vi "NI 5751 Multi Record Digital Trigger (Host).vi"() -> ()   [LabVIEW 2012] (continued)
2288.0, 5312.0, 7920.0, 9952.0, 11504.0, 12448.0, 12720.0, 12336.0, 11280.0, 9504.0, 7168.0, 4416.0, 1376.0, -1792.0, -4880.0, -7664.0, -9616.0, -10800.0, -11632.0, -12320.0, -12768.0, -12640.0, -11440.0, -9376.0, -6912.0, -4064.0, -1008.0, 2080.0, 5088.0, 7728.0, 9840.0, 11408.0, 12416.0, 12720.0, 12416.0, 11408.0, 9664.0, 7376.0, 4624.0, 1664.0, -1520.0, -4624.0, -7456.0, -9456.0, -10688.0, -11552.0, -12272.0, -12736.0, -12688.0, -11648.0, -9616.0, -7104.0, -4320.0, -1296.0, 1792.0, 4848.0, 7488.0, 9648.0, 11248.0, 12320.0, 12704.0, 12432.0, 11472.0, 9824.0, 7584.0, 4864.0, 1904.0, -1216.0, -4368.0, -7248.0, -9360.0, -10640.0, -11504.0, -12224.0, -12704.0, -12704.0, -11648.0, -9680.0, -7248.0, -4496.0, -1472.0, 1648.0, 4688.0, 7392.0, 9568.0, 11216.0, 12320.0, 12704.0, 12496.0, 11584.0, 9952.0, 7744.0, 5024.0, 2064.0, -1072.0, -4208.0, -7120.0, -9264.0]}, {"absoluteInitialX"=0.0, "xIncrement"=1.0, "wfm"=[-4672.0, -1712.0, 1376.0, 4464.0, 7184.0, 9392.0, 11088.0, 12240.0, 12720.0, 12528.0, 11696.0, 10128.0, 7984.0, 5360.0, 2400.0, -720.0, -3872.0, -6848.0, -9072.0, -10432.0, -11344.0, -12096.0, -12656.0, -12768.0, -11952.0, -10144.0, -7712.0, -4928.0, -1984.0, 1104.0, 4160.0, 6960.0, 9200.0, 10944.0, 12160.0, 12704.0, 12576.0, 11792.0, 10288.0, 8112.0, 5552.0, 2592.0, -528.0, -3664.0, -6672.0, -8976.0, -10384.0, -11312.0, -12048.0, -12624.0, -12768.0, -12032.0, -10224.0, -7792.0, -5072.0, -2128.0, 944.0, 4048.0, 6880.0, 9120.0, 10928.0, 12144.0, 12704.0, 12608.0, 11856.0, 10384.0, 8240.0, 5744.0, 2848.0, -288.0, -3472.0, -6512.0, -8832.0, -10304.0, -11248.0, -12000.0, -12576.0, -12752.0, -12096.0, -10336.0, -7968.0, -5248.0, -2352.0, 736.0, 3824.0, 6672.0, 9008.0, 10800.0, 12080.0, 12704.0, 12704.0, 12064.0, 10656.0, 8640.0, 6096.0, 3168.0, 112.0, -2992.0, -6032.0, -8528.0]}, {"absoluteInitialX"=0.0, "xIncrement"=1.0, "wfm"=[-2768.0, 272.0, 3392.0, 6288.0, 8672.0, 10576.0, 11920.0, 12688.0, 12720.0, 12128.0, 10848.0, 8896.0, 6416.0, 3584.0, 480.0, -2688.0, -5760.0, -8320.0, -9984.0, -11008.0, -11792.0, -12448.0, -12736.0, -12320.0, -10816.0, -8576.0, -5888.0, -2976.0, 32.0, 3088.0, 6048.0, 8512.0, 10448.0, 11872.0, 12624.0, 12736.0, 12176.0, 10944.0, 8960.0, 6544.0, 3712.0, 592.0, -2496.0, -5600.0, -8240.0, -9920.0, -10976.0, -11760.0, -12432.0, -12752.0, -12400.0, -10928.0, -8720.0, -6096.0, -3232.0, -224.0, 2928.0, 5904.0, 8400.0, 10320.0, 11760.0, 12576.0, 12768.0, 12256.0, 11056.0, 9136.0, 6704.0, 3920.0, 832.0, -2320.0, -5392.0, -8096.0, -9824.0, -10912.0, -11744.0, -12400.0, -12752.0, -12464.0, -11088.0, -8928.0, -6272.0, -3408.0, -416.0, 2720.0, 5728.0, 8208.0, 10224.0, 11680.0, 12576.0, 12768.0, 12336.0, 11216.0, 9376.0, 7008.0, 4240.0, 1216.0, -2016.0, -5072.0, -7824.0, -9664.0]}, {"absoluteInitialX"=0.0, "xIncrement"=1.0, "wfm"=[-3632.0, -624.0, 2480.0, 5488.0, 8080.0, 10128.0, 11616.0, 12560.0, 12800.0, 12368.0, 11280.0, 9504.0, 7120.0, 4416.0, 1376.0, -1776.0, -4864.0, -7712.0, -9584.0, -10752.0, -11584.0, -12272.0, -12688.0, -12560.0, -11360.0, -9296.0, -6736.0, -3888.0, -864.0, 2224.0, 5280.0, 7888.0, 9968.0, 11504.0, 12496.0, 12768.0, 12416.0, 11376.0, 9664.0, 7280.0, 4592.0, 1536.0, -1600.0, -4704.0, -7536.0, -9504.0, -10704.0, -11520.0, -12240.0, -12688.0, -12608.0, -11456.0, -9456.0, -6896.0, -4064.0, -1056.0, 2064.0, 5088.0, 7664.0, 9776.0, 11408.0, 12432.0, 12768.0, 12448.0, 11424.0, 9744.0, 7456.0, 4768.0, 1776.0, -1344.0, -4512.0, -7360.0, -9392.0, -10656.0, -11504.0, -12224.0, -12672.0, -12656.0, -11600.0, -9600.0, -7056.0, -4272.0, -1264.0, 1808.0, 4848.0, 7552.0, 9680.0, 11312.0, 12400.0, 12752.0, 12480.0, 11520.0, 9824.0, 7520.0, 4848.0, 1904.0, -1280.0, -4416.0, -7280.0, -9328.0]}, {"absoluteInitialX"=0.0, "xIncrement"=1.0, "wfm"=[-4400.0, -1424.0, 1712.0, 4720.0, 7408.0, 9600.0, 11248.0, 12320.0, 12736.0, 12528.0, 11568.0, 9968.0, 7760.0, 5056.0, 2096.0, -1040.0, -4192.0, -7120.0, -9264.0, -10544.0, -11424.0, -12176.0, -12672.0, -12704.0, -11792.0, -9920.0, -7440.0, -4672.0, -1696.0, 1392.0, 4416.0, 7184.0, 9440.0, 11136.0, 12240.0, 12704.0, 12528.0, 11648.0, 10064.0, 7904.0, 5248.0, 2256.0, -832.0, -4000.0, -6928.0, -9152.0, -10512.0, -11392.0, -12128.0, -12656.0, -12752.0, -11872.0, -10000.0, -7552.0, -4800.0, -1808.0, 1280.0, 4288.0, 7088.0, 9312.0, 11040.0, 12224.0, 12704.0, 12544.0, 11712.0, 10176.0, 8032.0, 5360.0, 2448.0, -656.0, -3792.0, -6768.0, -9040.0, -10432.0, -11344.0, -12112.0, -12656.0, -12768.0, -12016.0, -10192.0, -7792.0, -5040.0, -2096.0, 976.0, 4048.0, 6912.0, 9152.0, 10896.0, 12144.0, 12720.0, 12608.0, 11856.0, 10384.0, 8208.0, 5648.0, 2752.0, -320.0, -3520.0, -6544.0, -8880.0]}, {"absoluteInitialX"=0.0, "xIncrement"=1.0, "wfm"=[-2336.0, 720.0, 3824.0, 6672.0, 8976.0, 10784.0, 12064.0, 12672.0, 12624.0, 11952.0, 10480.0, 8432.0, 5840.0, 2944.0, -112.0, -3296.0, -6304.0, -8720.0, -10256.0, -11216.0, -11984.0, -12560.0, -12800.0, -12224.0, -10528.0, -8192.0, -5504.0, -2576.0, 448.0, 3520.0, 6448.0, 8800.0, 10640.0, 11968.0, 12656.0, 12624.0, 11984.0, 10624.0, 8608.0, 6064.0, 3216.0, 128.0, -3088.0, -6064.0, -8544.0, -10144.0, -11152.0, -11936.0, -12544.0, -12816.0, -12304.0, -10720.0, -8400.0, -5744.0, -2816.0, 192.0, 3296.0, 6192.0, 8624.0, 10512.0, 11888.0, 12608.0, 12688.0, 12096.0, 10800.0, 8832.0, 6400.0, 3568.0, 480.0, -2672.0, -5824.0, -8368.0, -10016.0, -11040.0, -11856.0, -12480.0, -12800.0, -12400.0, -10880.0, -8688.0, -6016.0, -3104.0, -96.0, 3024.0, 5984.0, 8432.0, 10368.0, 11808.0, 12592.0, 12704.0, 12192.0, 10944.0, 9040.0, 6592.0, 3840.0, 768.0, -2416.0, -5504.0, -8160.0, -9904.0]}, {"absoluteInitialX"=0.0, "xIncrement"=1.0, "wfm"=[-3296.0, -288.0, 2784.0, 5728.0, 8224.0, 10224.0, 11696.0, 12576.0, 12720.0, 12224.0, 11040.0, 9200.0, 6800.0, 3968.0, 912.0, -2224.0, -5264.0, -8000.0, -9808.0, -10896.0, -11712.0, -12384.0, -12784.0, -12528.0, -11200.0, -9024.0, -6416.0, -3552.0, -544.0, 2592.0, 5616.0, 8144.0, 10112.0, 11600.0, 12512.0, 12736.0, 12288.0, 11168.0, 9376.0, 6976.0, 4240.0, 1216.0, -1968.0, -5072.0, -7840.0, -9696.0, -10832.0, -11664.0, -12336.0, -12768.0, -12576.0, -11264.0, -9184.0, -6688.0, -3824.0, -800.0, 2352.0, 5408.0, 7936.0, 9968.0, 11520.0, 12448.0, 12704.0, 12352.0, 11248.0, 9488.0, 7216.0, 4464.0, 1440.0, -1680.0, -4816.0, -7632.0, -9568.0, -10752.0, -11600.0, -12288.0, -12736.0, -12640.0, -11456.0, -9392.0, -6864.0, -4048.0, -1008.0, 2048.0, 5056.0, 7712.0, 9840.0, 11408.0, 12448.0, 12720.0, 12384.0, 11408.0, 9712.0, 7392.0, 4672.0, 1680.0, -1456.0, -4592.0, -7424.0, -9440.0]}, {"absoluteInitialX"=0.0, "xIncrement"=1.0, "wfm"=[-4272.0, -1264.0, 1808.0, 4816.0, 7520.0, 9680.0, 11280.0, 12352.0, 12704.0, 12464.0, 11520.0, 9840.0, 7600.0, 4944.0, 1920.0, -1184.0, -4352.0, -7232.0, -9296.0, -10608.0, -11472.0, -12192.0, -12704.0, -12720.0, -11744.0, -9808.0, -7344.0, -4528.0, -1568.0, 1520.0, 4592.0, 7344.0, 9520.0, 11168.0, 12288.0, 12720.0, 12496.0, 11600.0, 9984.0, 7744.0, 5088.0, 2128.0, -976.0, -4112.0, -7040.0, -9216.0, -10544.0, -11440.0, -12176.0, -12688.0, -12768.0, -11904.0, -9952.0, -7552.0, -4768.0, -1808.0, 1328.0, 4384.0, 7104.0, 9328.0, 11024.0, 12208.0, 12688.0, 12512.0, 11680.0, 10128.0, 7968.0, 5296.0, 2384.0, -752.0, -3872.0, -6832.0, -9072.0, -10464.0, -11392.0, -12128.0, -12640.0, -12800.0, -11984.0, -10128.0, -7728.0, -5008.0, -2048.0, 1040.0, 4128.0, 6928.0, 9200.0, 10944.0, 12144.0, 12704.0, 12592.0, 11808.0, 10304.0, 8176.0, 5616.0, 2704.0, -400.0, -3552.0, -6592.0, -8912.0]}, {"absoluteInitialX"=0.0, "xIncrement"=1.0, "wfm"=[-2336.0, 656.0, 3776.0, 6640.0, 8976.0, 10784.0, 12032.0, 12656.0, 12608.0, 11888.0, 10512.0, 8448.0, 5856.0, 2992.0, -96.0, -3248.0, -6256.0, -8704.0, -10240.0, -11216.0, -11984.0, -12576.0, -12784.0, -12208.0, -10560.0, -8240.0, -5552.0, -2624.0, 448.0, 3552.0, 6496.0, 8832.0, 10672.0, 11968.0, 12640.0, 12656.0, 11984.0, 10592.0, 8544.0, 6064.0, 3184.0, 80.0, -3024.0, -6064.0, -8608.0, -10160.0, -11152.0, -11904.0, -12528.0, -12800.0, -12320.0, -10704.0, -8432.0, -5744.0, -2800.0, 272.0, 3392.0, 6288.0, 8640.0, 10528.0, 11904.0, 12624.0, 12672.0, 12112.0, 10832.0, 8832.0, 6352.0, 3488.0, 400.0, -2752.0, -5776.0, -8368.0, -10032.0, -11072.0, -11856.0, -12464.0, -12800.0, -12400.0, -10928.0, -8688.0, -6032.0, -3136.0, -96.0, 3008.0, 5984.0, 8416.0, 10368.0, 11792.0, 12560.0, 12672.0, 12160.0, 10944.0, 9024.0, 6576.0, 3760.0, 704.0, -2496.0, -5568.0, -8224.0, -9952.0]}, {"absoluteInitialX"=0.0, "xIncrement"=1.0, "wfm"=[-3376.0, -336.0, 2816.0, 5744.0, 8272.0, 10256.0, 11696.0, 12560.0, 12704.0, 12240.0, 11056.0, 9200.0, 6736.0, 4000.0, 944.0, -2208.0, -5328.0, -8048.0, -9840.0, -10912.0, -11728.0, -12400.0, -12800.0, -12544.0, -11200.0, -9056.0, -6464.0, -3600.0, -544.0, 2528.0, 5536.0, 8064.0, 10112.0, 11600.0, 12496.0, 12704.0, 12288.0, 11200.0, 9392.0, 7040.0, 4256.0, 1280.0, -1920.0, -5024.0, -7792.0, -9664.0, -10800.0, -11664.0, -12352.0, -12768.0, -12608.0, -11328.0, -9200.0, -6624.0, -3808.0, -768.0, 2288.0, 5296.0, 7872.0, 9952.0, 11536.0, 12480.0, 12752.0, 12384.0, 11312.0, 9552.0, 7200.0, 4480.0, 1472.0, -1632.0, -4832.0, -7648.0, -9584.0, -10752.0, -11600.0, -12288.0, -12736.0, -12624.0, -11472.0, -9424.0, -6848.0, -4016.0, -1008.0, 2112.0, 5120.0, 7760.0, 9872.0, 11424.0, 12432.0, 12752.0, 12384.0, 11344.0, 9632.0, 7280.0, 4560.0, 1584.0, -1568.0, -4704.0, -7552.0, -9504.0]}, {"absoluteInitialX"=0.0, "xIncrement"=1.0, "wfm"=[-4032.0, -1104.0, 1968.0, 4976.0, 7632.0, 9776.0, 11360.0, 12400.0, 12720.0, 12384.0, 11376.0, 9680.0, 7392.0, 4672.0, 1712.0, -1456.0, -4560.0, -7440.0, -9472.0, -10688.0, -11552.0, -12256.0, -12720.0, -12704.0, -11632.0, -9632.0, -7120.0, -4288.0, -1280.0, 1776.0, 4816.0, 7536.0, 9648.0, 11264.0, 12352.0, 12704.0, 12448.0, 11504.0, 9888.0, 7664.0, 4992.0, 1984.0, -1152.0, -4240.0, -7168.0, -9296.0, -10592.0, -11472.0, -12192.0, -12688.0, -12736.0, -11760.0, -9776.0, -7360.0, -4544.0, -1616.0, 1504.0, 4560.0, 7248.0, 9472.0, 11120.0, 12288.0, 12688.0, 12496.0, 11616.0, 10000.0, 7792.0, 5136.0, 2176.0, -1008.0, -4128.0, -7056.0, -9216.0, -10560.0, -11440.0, -12160.0, -12688.0, -12736.0, -11840.0, -9984.0, -7520.0, -4736.0, -1808.0, 1280.0, 4368.0, 7136.0, 9360.0, 11088.0, 12224.0, 12688.0, 12528.0, 11712.0, 10144.0, 8032.0, 5392.0, 2368.0, -768.0, -3904.0, -6832.0, -9072.0]}, {"absoluteInitialX"=0.0, "xIncrement"=1.0, "wfm"=[-2000.0, 1120.0, 4176.0, 6960.0, 9216.0, 10960.0, 12176.0, 12720.0, 12576.0, 11808.0, 10336.0, 8240.0, 5568.0, 2656.0, -464.0, -3600.0, -6608.0, -8912.0, -10336.0, -11280.0, -12048.0, -12608.0, -12768.0, -12048.0, -10272.0, -7888.0, -5184.0, -2208.0, 864.0, 3952.0, 6784.0, 9088.0, 10832.0, 12096.0, 12640.0, 12592.0, 11856.0, 10384.0, 8288.0, 5744.0, 2848.0, -272.0, -3424.0, -6448.0, -8816.0, -10304.0, -11248.0, -12000.0, -12608.0, -12800.0, -12160.0, -10448.0, -8112.0, -5408.0, -2448.0, 608.0, 3712.0, 6560.0, 8880.0, 10736.0, 12016.0, 12672.0, 12640.0, 11984.0, 10608.0, 8528.0, 6000.0, 3184.0, 112.0, -3088.0, -6144.0, -8592.0, -10160.0, -11152.0, -11920.0, -12528.0, -12816.0, -12288.0, -10688.0, -8416.0, -5696.0, -2784.0, 272.0, 3360.0, 6304.0, 8688.0, 10544.0, 11920.0, 12624.0, 12672.0, 12096.0, 10800.0, 8848.0, 6384.0, 3536.0, 480.0, -2704.0, -5760.0, -8336.0, -10016.0]}, {"absoluteInitialX"=0.0, "xIncrement"=1.0, "wfm"=[-3152.0, -112.0, 3056.0, 5968.0, 8400.0, 10384.0, 11776.0, 12576.0, 12688.0, 12160.0, 10928.0, 9056.0, 6576.0, 3744.0, 640.0, -2480.0, -5584.0, -8224.0, -9920.0, -10976.0, -11776.0, -12432.0, -12800.0, -12496.0, -11072.0, -8864.0, -6256.0, -3392.0, -368.0, 2768.0, 5744.0, 8288.0, 10240.0, 11664.0, 12544.0, 12688.0, 12208.0, 11024.0, 9104.0, 6688.0, 3936.0, 880.0, -2304.0, -5376.0, -8048.0, -9856.0, -10928.0, -11744.0, -12432.0, -12816.0, -12544.0, -11232.0, -9104.0, -6464.0, -3584.0, -576.0, 2528.0, 5520.0, 8048.0, 10080.0, 11584.0, 12496.0, 12704.0, 12288.0, 11152.0, 9328.0, 6976.0, 4144.0, 1120.0, -1984.0, -5104.0, -7872.0, -9728.0, -10864.0, -11696.0, -12368.0, -12800.0, -12608.0, -11376.0, -9232.0, -6672.0, -3856.0, -848.0, 2240.0, 5264.0, 7856.0, 9920.0, 11456.0, 12416.0, 12688.0, 12320.0, 11232.0, 9520.0, 7168.0, 4400.0, 1408.0, -1696.0, -4800.0, -7632.0, -9600.0]}, {"absoluteInitialX"=0.0, "xIncrement"=1.0, "wfm"=[-4080.0, -1056.0, 2048.0, 5056.0, 7696.0, 9840.0, 11392.0, 12400.0, 12704.0, 12368.0, 11360.0, 9648.0, 7344.0, 4624.0, 1616.0, -1504.0, -4672.0, -7504.0, -9504.0, -10704.0, -11584.0, -12288.0, -12752.0, -12704.0, -11616.0, -9632.0, -7120.0, -4240.0, -1248.0, 1840.0, 4848.0, 7520.0, 9664.0, 11264.0, 12336.0, 12720.0, 12432.0, 11440.0, 9760.0, 7504.0, 4800.0, 1808.0, -1280.0, -4416.0, -7360.0, -9376.0, -10640.0, -11536.0, -12256.0, -12752.0, -12736.0, -11712.0, -9760.0, -7280.0, -4480.0, -1488.0, 1584.0, 4608.0, 7328.0, 9504.0, 11152.0, 12288.0, 12736.0, 12496.0, 11584.0, 10016.0, 7840.0, 5168.0, 2224.0, -960.0, -4128.0, -7040.0, -9184.0, -10528.0, -11408.0, -12160.0, -12688.0, -12768.0, -11856.0, -9968.0, -7504.0, -4688.0, -1728.0, 1344.0, 4400.0, 7200.0, 9376.0, 11056.0, 12240.0, 12720.0, 12528.0, 11728.0, 10176.0, 7984.0, 5344.0, 2432.0, -624.0, -3808.0, -6784.0, -9024.0]}, {"absoluteInitialX"=0.0, "xIncrement"=1.0, "wfm"=[-2016.0, 1008.0, 4096.0, 6880.0, 9168.0, 10928.0, 12160.0, 12736.0, 12640.0, 11904.0, 10496.0, 8416.0, 5808.0, 2896.0, -208.0, -3344.0, -6352.0, -8768.0, -10256.0, -11184.0, -11952.0, -12544.0, -12752.0, -12128.0, -10464.0, -8128.0, -5424.0, -2528.0, 608.0, 3680.0, 6544.0, 8880.0, 10736.0, 12016.0, 12704.0, 12672.0, 12016.0, 10656.0, 8592.0, 6080.0, 3216.0, 128.0, -3024.0, -6032.0, -8544.0, -10128.0, -11104.0, -11904.0, -12512.0, -12752.0, -12208.0, -10624.0, -8320.0, -5632.0, -2704.0, 320.0, 3424.0, 6336.0, 8752.0, 10608.0, 11936.0, 12688.0, 12704.0, 12096.0, 10752.0, 8784.0, 6352.0, 3456.0, 336.0, -2816.0, -5824.0, -8368.0, -10032.0, -11056.0, -11824.0, -12464.0, -12784.0, -12336.0, -10832.0, -8528.0, -5904.0, -3008.0, 16.0, 3168.0, 6080.0, 8544.0, 10448.0, 11856.0, 12624.0, 12720.0, 12176.0, 10880.0, 8960.0, 6512.0, 3648.0, 544.0, -2592.0, -5664.0, -8288.0, -9968.0]}, {"absoluteInitialX"=0.0, "xIncrement"=1.0, "wfm"=[-3136.0, -160.0, 2944.0, 5936.0, 8416.0, 10352.0, 11776.0, 12608.0, 12720.0, 12208.0, 10960.0, 9056.0, 6608.0, 3808.0, 752.0, -2416.0, -5504.0, -8144.0, -9904.0, -10976.0, -11776.0, -12400.0, -12784.0, -12432.0, -11008.0, -8848.0, -6192.0, -3296.0, -272.0, 2848.0, 5792.0, 8256.0, 10272.0, 11712.0, 12560.0, 12736.0, 12272.0, 11072.0, 9232.0, 6832.0, 4016.0, 992.0, -2176.0, -5264.0, -7968.0, -9776.0, -10880.0, -11680.0, -12368.0, -12768.0, -12544.0, -11216.0, -9088.0, -6496.0, -3632.0, -608.0, 2512.0, 5488.0, 8064.0, 10096.0, 11616.0, 12528.0, 12704.0, 12272.0, 11216.0, 9424.0, 7056.0, 4272.0, 1248.0, -1936.0, -5008.0, -7792.0, -9648.0, -10816.0, -11632.0, -12336.0, -12752.0, -12576.0, -11328.0, -9280.0, -6688.0, -3808.0, -800.0, 2304.0, 5280.0, 7872.0, 9984.0, 11504.0, 12480.0, 12704.0, 12336.0, 11264.0, 9488.0, 7104.0, 4368.0, 1360.0, -1840.0, -4960.0, -7712.0, -9648.0]}, {"absoluteInitialX"=0.0, "xIncrement"=1.0, "wfm"=[-3968.0, -944.0, 2144.0, 5152.0, 7776.0, 9856.0, 11424.0, 12432.0, 12720.0, 12368.0, 11328.0, 9568.0, 7280.0, 4576.0, 1568.0, -1568.0, -4704.0, -7520.0, -9520.0, -10752.0, -11584.0, -12288.0, -12752.0, -12688.0, -11552.0, -9504.0, -7024.0, -4240.0, -1216.0, 1920.0, 4944.0, 7600.0, 9728.0, 11344.0, 12368.0, 12720.0, 12432.0, 11424.0, 9744.0, 7488.0, 4800.0, 1824.0, -1360.0, -4480.0, -7344.0, -9408.0, -10656.0, -11520.0, -12224.0, -12720.0, -12704.0, -11664.0, -9696.0, -7232.0, -4416.0, -1392.0, 1680.0, 4704.0, 7376.0, 9552.0, 11248.0, 12336.0, 12736.0, 12464.0, 11552.0, 9904.0, 7712.0, 5056.0, 2080.0, -1088.0, -4208.0, -7120.0, -9280.0, -10576.0, -11456.0, -12160.0, -12688.0, -12752.0, -11824.0, -9920.0, -7440.0, -4704.0, -1728.0, 1376.0, 4448.0, 7152.0, 9376.0, 11104.0, 12240.0, 12704.0, 12544.0, 11632.0, 10048.0, 7872.0, 5168.0, 2240.0, -848.0, -4016.0, -6992.0, -9184.0]}, {"absoluteInitialX"=0.0, "xIncrement"=1.0, "wfm"=[-4912.0, -1920.0, 1168.0, 4224.0, 7040.0, 9280.0, 10992.0, 12192.0, 12656.0, 12528.0, 11728.0, 10208.0, 8064.0, 5408.0, 2480.0, -640.0, -3776.0, -6720.0, -9024.0, -10448.0, -11328.0, -12112.0, -12656.0, -12800.0, -12016.0, -10176.0, -7824.0, -5040.0, -2064.0, 976.0, 4032.0, 6896.0, 9184.0, 10928.0, 12128.0, 12656.0, 12544.0, 11744.0, 10304.0, 8112.0, 5504.0, 2560.0, -528.0, -3664.0, -6656.0, -8992.0, -10400.0, -11312.0, -12080.0, -12640.0, -12784.0, -12064.0, -10272.0, -7888.0, -5168.0, -2208.0, 864.0, 3936.0, 6752.0, 9088.0, 10832.0, 12080.0, 12656.0, 12560.0, 11824.0, 10352.0, 8256.0, 5664.0, 2768.0, -416.0, -3536.0, -6528.0, -8864.0, -10352.0, -11296.0, -12048.0, -12608.0, -12800.0, -12144.0, -10384.0, -8032.0, -5280.0, -2336.0, 736.0, 3824.0, 6640.0, 8944.0, 10768.0, 12048.0, 12672.0, 12640.0, 11968.0, 10608.0, 8544.0, 5952.0, 3120.0, 32.0, -3120.0, -6192.0, -8656.0]}, {"absoluteInitialX"=0.0, "xIncrement"=1.0, "wfm"=[-2672.0, 368.0, 3472.0, 6352.0, 8736.0, 10656.0, 11968.0, 12672.0, 12672.0, 12112.0, 10816.0, 8720.0, 6240.0, 3440.0, 352.0, -2752.0, -5840.0, -8400.0, -10032.0, -11040.0, -11840.0, -12448.0, -12768.0, -12320.0, -10784.0, -8592.0, -5904.0, -2992.0, 48.0, 3120.0, 6064.0, 8512.0, 10448.0, 11824.0, 12608.0, 12672.0, 12144.0, 10880.0, 8960.0, 6512.0, 3632.0, 544.0, -2688.0, -5728.0, -8304.0, -9984.0, -11024.0, -11808.0, -12448.0, -12784.0, -12400.0, -10912.0, -8704.0, -6032.0, -3168.0, -144.0, 2928.0, 5888.0, 8368.0, 10320.0, 11744.0, 12576.0, 12752.0, 12272.0, 11040.0, 9168.0, 6784.0, 3968.0, 896.0, -2240.0, -5344.0, -8064.0, -9824.0, -10912.0, -11728.0, -12384.0, -12768.0, -12480.0, -11152.0, -8992.0, -6352.0, -3472.0, -464.0, 2672.0, 5600.0, 8160.0, 10160.0, 11664.0, 12544.0, 12752.0, 12288.0, 11120.0, 9328.0, 6912.0, 4112.0, 1088.0, -1984.0, -5136.0, -7872.0, -9712.0]}, {"absoluteInitialX"=0.0, "xIncrement"=1.0, "wfm"=[-3680.0, -656.0, 2464.0, 5408.0, 7984.0, 10064.0, 11568.0, 12544.0, 12752.0, 12384.0, 11248.0, 9456.0, 7120.0, 4320.0, 1312.0, -1824.0, -4976.0, -7760.0, -9648.0, -10784.0, -11616.0, -12320.0, -12752.0, -12624.0, -11408.0, -9296.0, -6784.0, -3984.0, -960.0, 2176.0, 5168.0, 7824.0, 9920.0, 11440.0, 12432.0, 12720.0, 12352.0, 11328.0, 9552.0, 7216.0, 4512.0, 1472.0, -1616.0, -4752.0, -7632.0, -9536.0, -10736.0, -11584.0, -12288.0, -12736.0, -12672.0, -11520.0, -9456.0, -6928.0, -4144.0, -1152.0, 1968.0, 5024.0, 7632.0, 9776.0, 11344.0, 12384.0, 12736.0, 12416.0, 11408.0, 9744.0, 7440.0, 4688.0, 1680.0, -1440.0, -4592.0, -7440.0, -9440.0, -10688.0, -11536.0, -12240.0, -12720.0, -12688.0, -11632.0, -9632.0, -7136.0, -4336.0, -1360.0, 1760.0, 4784.0, 7488.0, 9648.0, 11232.0, 12352.0, 12704.0, 12416.0, 11456.0, 9792.0, 7520.0, 4816.0, 1856.0, -1280.0, -4416.0, -7296.0, -9376.0]}, {"absoluteInitialX"=0.0, "xIncrement"=1.0, "wfm"=[-4464.0, -1504.0, 1616.0, 4656.0, 7344.0, 9552.0, 11184.0, 12304.0, 12704.0, 12464.0, 11504.0, 9840.0, 7616.0, 5024.0, 2000.0, -1152.0, -4288.0, -7184.0, -9312.0, -10576.0, -11472.0, -12192.0, -12704.0, -12736.0, -11792.0, -9840.0, -7392.0, -4592.0, -1616.0, 1488.0, 4528.0, 7232.0, 9424.0, 11136.0, 12256.0, 12704.0, 12512.0, 11648.0, 10048.0, 7888.0, 5168.0, 2176.0, -944.0, -4048.0, -6976.0, -9184.0, -10512.0, -11392.0, -12144.0, -12672.0, -12768.0, -11888.0, -10032.0, -7648.0, -4880.0, -1840.0, 1248.0, 4288.0, 7088.0, 9312.0, 11024.0, 12208.0, 12688.0, 12544.0, 11712.0, 10192.0, 8016.0, 5456.0, 2512.0, -656.0, -3792.0, -6736.0, -9008.0, -10400.0, -11344.0, -12112.0, -12624.0, -12752.0, -12000.0, -10160.0, -7744.0, -5008.0, -2080.0, 960.0, 4064.0, 6880.0, 9184.0, 10944.0, 12144.0, 12704.0, 12624.0, 11888.0, 10448.0, 8336.0, 5760.0, 2816.0, -288.0, -3424.0, -6416.0, -8784.0]}, {"absoluteInitialX"=0.0, "xIncrement"=1.0, "wfm"=[-2384.0, 656.0, 3728.0, 6624.0, 8928.0, 10736.0, 12048.0, 12720.0, 12688.0, 12032.0, 10640.0, 8608.0, 6080.0, 3248.0, 176.0, -3024.0, -6032.0, -8528.0, -10112.0, -11104.0, -11856.0, -12496.0, -12736.0, -12240.0, -10640.0, -8320.0, -5648.0, -2784.0, 272.0, 3376.0, 6288.0, 8704.0, 10576.0, 11936.0, 12688.0, 12736.0, 12096.0, 10832.0, 8816.0, 6352.0, 3504.0, 416.0, -2736.0, -5840.0, -8368.0, -10000.0, -11008.0, -11808.0, -12448.0, -12752.0, -12304.0, -10800.0, -8560.0, -5856.0, -2976.0, 96.0, 3200.0, 6112.0, 8544.0, 10512.0, 11888.0, 12656.0, 12736.0, 12208.0, 10928.0, 9040.0, 6560.0, 3728.0, 672.0, -2512.0, -5584.0, -8192.0, -9888.0, -10944.0, -11760.0, -12400.0, -12736.0, -12400.0, -10960.0, -8736.0, -6128.0, -3232.0, -224.0, 2896.0, 5856.0, 8352.0, 10336.0, 11744.0, 12592.0, 12768.0, 12320.0, 11088.0, 9216.0, 6832.0, 4032.0, 944.0, -2192.0, -5328.0, -8016.0, -9792.0]}, {"absoluteInitialX"=0.0, "xIncrement"=1.0, "wfm"=[-3472.0, -464.0, 2688.0, 5664.0, 8160.0, 10192.0, 11664.0, 12576.0, 12752.0, 12272.0, 11104.0, 9280.0, 6864.0, 4096.0, 1024.0, -2144.0, -5216.0, -7920.0, -9744.0, -10848.0, -11648.0, -12352.0, -12736.0, -12512.0, -11184.0, -9040.0, -6464.0, -3648.0, -640.0, 2544.0, 5552.0, 8128.0, 10112.0, 11616.0, 12528.0, 12720.0, 12256.0, 11120.0, 9296.0, 6912.0, 4112.0, 1104.0, -2080.0, -5168.0, -7904.0, -9744.0, -10864.0, -11664.0, -12352.0, -12752.0, -12512.0, -11248.0, -9072.0, -6512.0, -3664.0, -592.0, 2512.0, 5472.0, 8016.0, 10080.0, 11584.0, 12528.0, 12736.0, 12336.0, 11200.0, 9392.0, 7024.0, 4176.0, 1184.0, -1952.0, -5056.0, -7776.0, -9664.0, -10800.0, -11664.0, -12336.0, -12752.0, -12560.0, -11296.0, -9216.0, -6640.0, -3776.0, -752.0, 2352.0, 5408.0, 7952.0, 10032.0, 11520.0, 12496.0, 12736.0, 12352.0, 11232.0, 9488.0, 7104.0, 4320.0, 1312.0, -1808.0, -4976.0, -7760.0, -9648.0]}, {"absoluteInitialX"=0.0, "xIncrement"=1.0, "wfm"=[-3888.0, -896.0, 2240.0, 5232.0, 7824.0, 9904.0, 11456.0, 12464.0, 12752.0, 12400.0, 11360.0, 9616.0, 7280.0, 4544.0, 1504.0, -1600.0, -4704.0, -7520.0, -9504.0, -10704.0, -11552.0, -12240.0, -12720.0, -12656.0, -11504.0, -9504.0, -6928.0, -4064.0, -1056.0, 2016.0, 5008.0, 7680.0, 9808.0, 11392.0, 12432.0, 12736.0, 12448.0, 11472.0, 9776.0, 7472.0, 4752.0, 1760.0, -1392.0, -4480.0, -7376.0, -9392.0, -10624.0, -11472.0, -12208.0, -12688.0, -12656.0, -11584.0, -9584.0, -7072.0, -4240.0, -1248.0, 1888.0, 4880.0, 7536.0, 9696.0, 11312.0, 12400.0, 12768.0, 12512.0, 11568.0, 9920.0, 7680.0, 4992.0, 2016.0, -1120.0, -4272.0, -7152.0, -9264.0, -10560.0, -11408.0, -12144.0, -12640.0, -12656.0, -11680.0, -9728.0, -7296.0, -4544.0, -1552.0, 1600.0, 4624.0, 7392.0, 9552.0, 11216.0, 12352.0, 12768.0, 12576.0, 11648.0, 10048.0, 7904.0, 5264.0, 2288.0, -864.0, -3952.0, -6896.0, -9104.0]}, {"absoluteInitialX"=0.0, "xIncrement"=1.0, "wfm"=[-4784.0, -1808.0, 1312.0, 4384.0, 7136.0, 9344.0, 11088.0, 12288.0, 12784.0, 12656.0, 11840.0, 10320.0, 8160.0, 5632.0, 2688.0, -448.0, -3568.0, -6592.0, -8864.0, -10304.0, -11232.0, -11952.0, -12560.0, -12704.0, -11984.0, -10208.0, -7808.0, -5056.0, -2144.0, 912.0, 4000.0, 6848.0, 9152.0, 10928.0, 12192.0, 12752.0, 12656.0, 11920.0, 10480.0, 8368.0, 5840.0, 2960.0, -144.0, -3280.0, -6336.0, -8736.0, -10208.0, -11184.0, -11952.0, -12512.0, -12736.0, -12080.0, -10416.0, -8016.0, -5280.0, -2368.0, 688.0, 3792.0, 6656.0, 8976.0, 10848.0, 12112.0, 12736.0, 12704.0, 12016.0, 10592.0, 8544.0, 5984.0, 3120.0, -32.0, -3152.0, -6160.0, -8608.0, -10160.0, -11104.0, -11904.0, -12496.0, -12720.0, -12160.0, -10496.0, -8160.0, -5488.0, -2592.0, 496.0, 3632.0, 6528.0, 8928.0, 10736.0, 12032.0, 12736.0, 12752.0, 12112.0, 10704.0, 8736.0, 6224.0, 3344.0, 272.0, -2912.0, -5920.0, -8448.0]}, {"absoluteInitialX"=0.0, "xIncrement"=1.0, "wfm"=[-2768.0, 288.0, 3392.0, 6336.0, 8736.0, 10592.0, 11952.0, 12688.0, 12752.0, 12144.0, 10816.0, 8848.0, 6352.0, 3456.0, 400.0, -2688.0, -5792.0, -8352.0, -9984.0, -10992.0, -11792.0, -12416.0, -12736.0, -12304.0, -10752.0, -8528.0, -5856.0, -2976.0, 48.0, 3168.0, 6112.0, 8560.0, 10496.0, 11888.0, 12656.0, 12736.0, 12192.0, 10928.0, 8992.0, 6544.0, 3712.0, 656.0, -2512.0, -5600.0, -8192.0, -9904.0, -10960.0, -11744.0, -12400.0, -12736.0, -12352.0, -10880.0, -8704.0, -6016.0, -3120.0, -96.0, 2992.0, 5968.0, 8448.0, 10400.0, 11824.0, 12640.0, 12784.0, 12304.0, 11104.0, 9184.0, 6736.0, 3952.0, 928.0, -2192.0, -5312.0, -8000.0, -9792.0, -10864.0, -11680.0, -12320.0, -12720.0, -12448.0, -11072.0, -8912.0, -6304.0, -3440.0, -416.0, 2720.0, 5728.0, 8208.0, 10240.0, 11712.0, 12608.0, 12784.0, 12352.0, 11232.0, 9408.0, 7008.0, 4256.0, 1216.0, -1968.0, -5072.0, -7808.0, -9632.0]}, {"absoluteInitialX"=0.0, "xIncrement"=1.0, "wfm"=[-3744.0, -752.0, 2368.0, 5392.0, 7968.0, 10016.0, 11568.0, 12528.0, 12768.0, 12384.0, 11328.0, 9568.0, 7232.0, 4464.0, 1472.0, -1712.0, -4800.0, -7648.0, -9520.0, -10720.0, -11568.0, -12256.0, -12704.0, -12592.0, -11408.0, -9312.0, -6832.0, -3984.0, -992.0, 2144.0, 5184.0, 7760.0, 9856.0, 11440.0, 12432.0, 12768.0, 12432.0, 11392.0, 9632.0, 7360.0, 4656.0, 1632.0, -1520.0, -4624.0, -7472.0, -9456.0, -10688.0, -11520.0, -12256.0, -12704.0, -12624.0, -11488.0, -9472.0, -6992.0, -4144.0, -1120.0, 1984.0, 4976.0, 7648.0, 9792.0, 11376.0, 12416.0, 12752.0, 12464.0, 11488.0, 9808.0, 7568.0, 4816.0, 1808.0, -1280.0, -4368.0, -7264.0, -9360.0, -10592.0, -11472.0, -12208.0, -12688.0, -12704.0, -11664.0, -9680.0, -7232.0, -4400.0, -1424.0, 1680.0, 4720.0, 7472.0, 9632.0, 11248.0, 12352.0, 12736.0, 12496.0, 11584.0, 9984.0, 7712.0, 5120.0, 2128.0, -992.0, -4144.0, -7072.0, -9216.0]}, {"absoluteInitialX"=0.0, "xIncrement"=1.0, "wfm"=[-4624.0, -1632.0, 1472.0, 4544.0, 7248.0, 9504.0, 11120.0, 12288.0, 12736.0, 12544.0, 11664.0, 10080.0, 7888.0, 5232.0, 2272.0, -816.0, -3936.0, -6896.0, -9152.0, -10480.0, -11376.0, -12128.0, -12640.0, -12736.0, -11872.0, -10016.0, -7552.0, -4832.0, -1856.0, 1232.0, 4304.0, 7136.0, 9328.0, 11040.0, 12240.0, 12720.0, 12560.0, 11744.0, 10224.0, 8032.0, 5360.0, 2480.0, -656.0, -3840.0, -6816.0, -9056.0, -10432.0, -11360.0, -12112.0, -12640.0, -12768.0, -11968.0, -10128.0, -7760.0, -4976.0, -1984.0, 1088.0, 4160.0, 6944.0, 9184.0, 10944.0, 12160.0, 12720.0, 12624.0, 11824.0, 10336.0, 8224.0, 5664.0, 2672.0, -448.0, -3584.0, -6544.0, -8896.0, -10336.0, -11280.0, -12048.0, -12592.0, -12784.0, -12080.0, -10304.0, -7904.0, -5184.0, -2256.0, 816.0, 3904.0, 6720.0, 9088.0, 10848.0, 12096.0, 12704.0, 12688.0, 11968.0, 10544.0, 8544.0, 5920.0, 3040.0, -48.0, -3216.0, -6256.0, -8672.0]}, {"absoluteInitialX"=0.0, "xIncrement"=1.0, "wfm"=[-2608.0, 464.0, 3536.0, 6480.0, 8816.0, 10688.0, 12000.0, 12704.0, 12688.0, 12080.0, 10720.0, 8752.0, 6208.0, 3328.0, 224.0, -2880.0, -5904.0, -8464.0, -10080.0, -11088.0, -11840.0, -12496.0, -12784.0, -12304.0, -10736.0, -8496.0, -5776.0, -2864.0, 192.0, 3344.0, 6256.0, 8656.0, 10544.0, 11904.0, 12640.0, 12688.0, 12080.0, 10784.0, 8832.0, 6336.0, 3504.0, 432.0, -2800.0, -5792.0, -8384.0, -10016.0, -11040.0, -11840.0, -12464.0, -12768.0, -12352.0, -10896.0, -8656.0, -5968.0, -3008.0, 0.0, 3088.0, 6016.0, 8448.0, 10416.0, 11808.0, 12624.0, 12720.0, 12192.0, 10960.0, 9040.0, 6608.0, 3760.0, 688.0, -2448.0, -5536.0, -8176.0, -9888.0, -10960.0, -11760.0, -12416.0, -12800.0, -12480.0, -11024.0, -8864.0, -6288.0, -3392.0, -304.0, 2816.0, 5760.0, 8256.0, 10240.0, 11696.0, 12576.0, 12704.0, 12240.0, 11040.0, 9168.0, 6752.0, 3952.0, 880.0, -2208.0, -5312.0, -8048.0, -9824.0]}, {"absoluteInitialX"=0.0, "xIncrement"=1.0, "wfm"=[-3664.0, -640.0, 2496.0, 5520.0, 8064.0, 10096.0, 11568.0, 12480.0, 12704.0, 12304.0, 11184.0, 9392.0, 7024.0, 4256.0, 1232.0, -1936.0, -5040.0, -7808.0, -9664.0, -10832.0, -11680.0, -12368.0, -12768.0, -12608.0, -11392.0, -9280.0, -6688.0, -3904.0, -944.0, 2208.0, 5232.0, 7856.0, 9920.0, 11472.0, 12416.0, 12688.0, 12336.0, 11264.0, 9536.0, 7200.0, 4400.0, 1392.0, -1728.0, -4800.0, -7600.0, -9600.0, -10784.0, -11616.0, -12320.0, -12752.0, -12656.0, -11520.0, -9488.0, -6976.0, -4128.0, -1136.0, 2016.0, 5040.0, 7664.0, 9776.0, 11360.0, 12368.0, 12688.0, 12384.0, 11408.0, 9696.0, 7440.0, 4656.0, 1680.0, -1408.0, -4576.0, -7440.0, -9456.0, -10704.0, -11552.0, -12288.0, -12752.0, -12720.0, -11632.0, -9664.0, -7168.0, -4352.0, -1392.0, 1696.0, 4784.0, 7472.0, 9600.0, 11248.0, 12320.0, 12688.0, 12432.0, 11504.0, 9808.0, 7552.0, 4912.0, 1904.0, -1248.0, -4336.0, -7248.0, -9360.0]}]
  in  "Trigger Channel":enum16{"DI 0", "DI 1"}(ring)
  in  "Trigger Type":enum16{"Immediate", "Digital"}(ring)
  in  "Num Records":u32=100
  in  "Num Samples":u32=100
  # "Trigger"
  # "Analog Input"
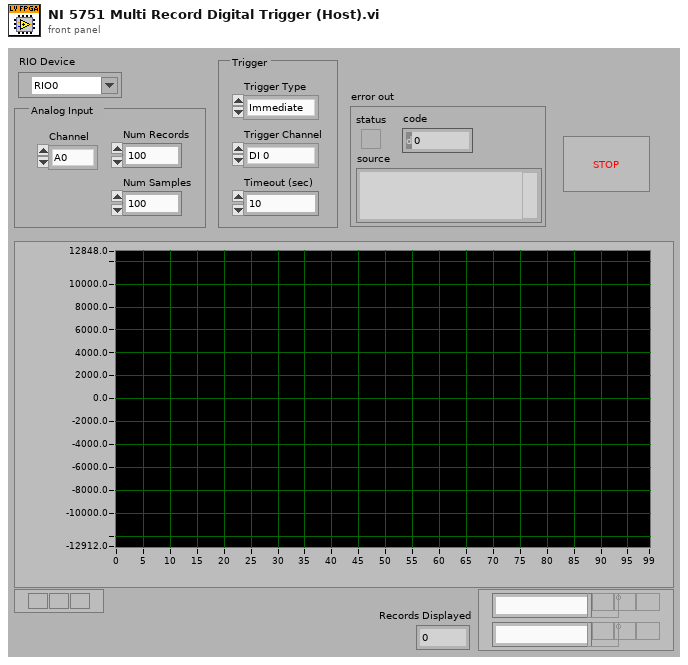
[diagram p1: front panel]
types:
  T1 = enum16{"A0", "A1", "A2", "A3", "A4", "A5", "A6", "A7", "B8", "B9", "B10", "B11", "B12", "B13", "B14", "B15"}
  T2 = typedef "nirio_resource_hc.ctl" = tag
  T3 = cluster{"absoluteInitialX":dbl, "xIncrement":dbl, "wfm":dbl[]}[]
  T4 = cluster{"absoluteInitialX":dbl, "xIncrement":dbl, "Data":void[]}
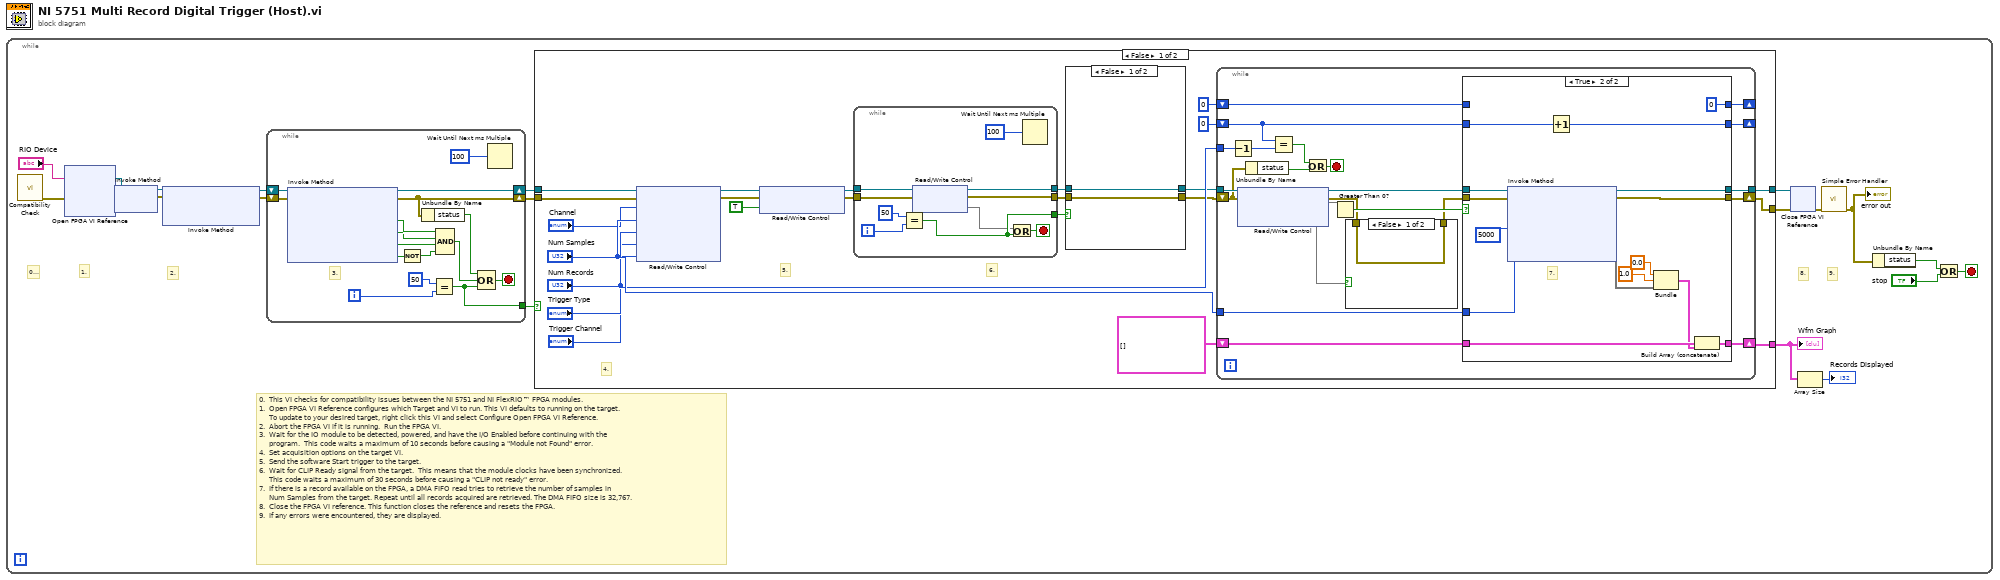
[diagram p0: block diagram]
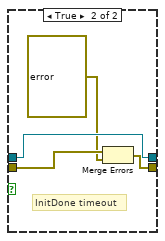
[diagram p2: hidden frame]
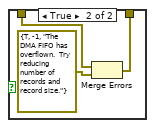
[diagram p3: hidden frame]
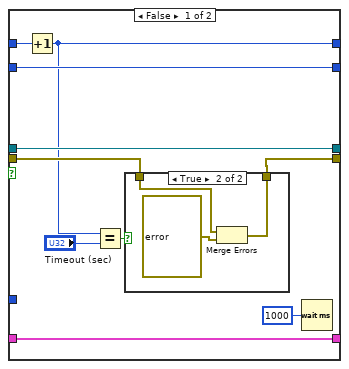
[diagram p4: hidden frame]
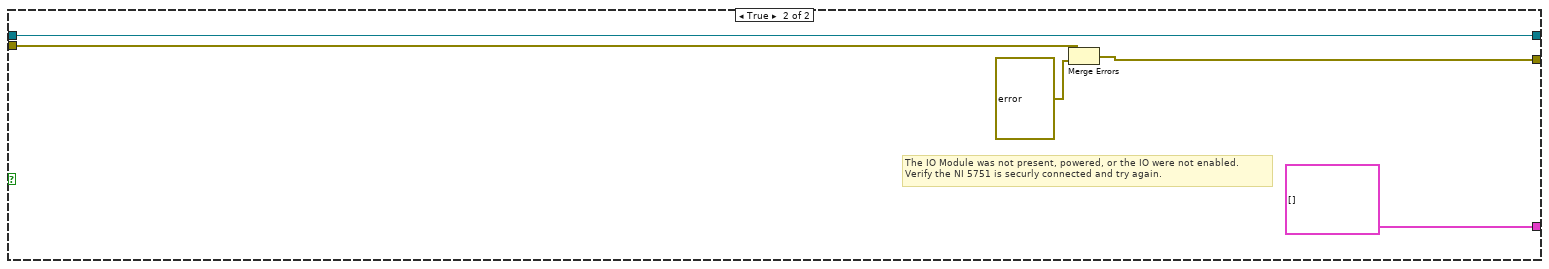
[diagram p6: hidden frame]
diagram:
  n1 = while {
    stop <- w5 stop-if-true
    # "1."
    # "0.0."
    # "2."
    # "9."
    # "8."
    # "0.  This VI checks for compatibility issues between the NI 5751 and NI FlexRIO™ FPGA modules. \n1.  Open FPGA VI Reference configures which Target and VI to run. This VI defaults to running on the target.  \n     To update to your desired target, right click this VI and select Configure Open FPGA VI Reference.\n2.  Abort the FPGA VI if it is running.  Run the FPGA VI. \n3.  Wait for the IO module to be detected, powered, and have the I/O Enabled before continuing with the \n     program.  This code waits a maximum of 10 seconds before causing a \"Module not Found\" error.\n4.  Set acquisition options on the target VI.\n5.  Send the software Start trigger to the target.\n6.  Wait for CLIP Ready signal from the target.  This means that the module clocks have been synchronized.  \n     This code waits a maximum of 30 seconds before causing a \"CLIP not ready\" error.\n7.  If there is a record available on the FPGA, a DMA FIFO read tries to retrieve the number of samples in \n     Num Samples from the target. Repeat until all records acquired are retrieved. The DMA FIFO size is 32,767.  \n8.  Close the FPGA VI reference. This function closes the reference and resets the FPGA.\n9.  If any errors were encountered, they are displayed."
    n2 = call "Compatibility Check.vi"() -> ("error out"=w1:errorcluster)  [unwired: 2 in, 9 out]
    n3 = xnode "Open FPGA VI Reference"("error in"=w1, "resource name"="RIO Device") -> ("FPGA VI Reference Out"=w10:refnum<k20>, "error out"=w9:errorcluster)
    n4 = xnode "Invoke Method"("FPGA VI Reference In"=w10, "error in"=w9) -> ("FPGA VI Reference Out"=w7:refnum<k20>, "error out"=w8:errorcluster)
    n5 = xnode "Invoke Method"("FPGA VI Reference In"=w7, "error in"=w8) -> ("FPGA VI Reference Out"=w12:refnum<k20>, "error out"=w11:errorcluster)  [unwired: 1 in]
    n6 = while {
      shift-right: [w126] -> w19
      shift-left: w11 -> [w134]
      shift-right: [w133] -> w16
      shift-left: w12 -> [w135]
      tunnel: [w122] -> w20
      i -> [w128]
      stop <- w123 stop-if-true
      # "3."
      n7 = xnode "Invoke Method"("FPGA VI Reference In"=w135, "error in"=w134) -> ("FPGA VI Reference Out"=w133:refnum<k20>, "error out"=w126:errorcluster, "IO Module Present?"=w132:bool, "Power Enabled?"=w131:bool, "IO Enabled?"=w130:bool, "IO Module Mismatch?"=w121:bool)
      n8 = Not(x=w121) -> (.not. x?=w120:bool)
      n9 = Unbundle By Name(w126) -> ("status"=w125:bool)
      n10 = Equal?(x=50, y=w128) -> (x = y?=w122:bool)
      n11 = Compound Arithmetic op=AND(w132, w131, w130, w120) -> (w124:bool)
      n12 = Compound Arithmetic op=OR(w125, w124, w122) -> (w123:bool)
      n13 = Wait Until Next ms Multiple(millisecond multiple=u32 100) -> ()  [unwired: 1 out]
    }
    n14 = case shown="False" w20 {
      tunnel: w19 -> [w40 w118]
      tunnel: [w42 w117] -> w17
      tunnel: [w43 w116] -> w15
      tunnel: w16 -> [w39 w116]
      tunnel: [w31 T3 []] -> w14
      frame False {
        # "6."
        # "5."
        # "4."
        n15 = xnode "Read/Write Control"("FPGA VI Reference In"=w39, "error in"=w40, "Read Channel"="Channel", "Num Samples"="Num Samples", "Num Records"="Num Records", "Trigger Type"="Trigger Type", "Trigger Channel"="Trigger Channel") -> ("FPGA VI Reference Out"=w38:refnum<k20>, "error out"=w37:errorcluster)
        n16 = xnode "Read/Write Control"("FPGA VI Reference In"=w38, "error in"=w37, "Start Acquisition"=TRUE) -> ("FPGA VI Reference Out"=w25:refnum<k20>, "error out"=w26:errorcluster)
        n17 = while {
          tunnel: w25 -> [w59]
          tunnel: [w55] -> w28
          tunnel: [w54] -> w27
          tunnel: [w52] -> w29
          tunnel: w26 -> [w50]
          i -> [w57]
          stop <- w53 stop-if-true
          n18 = Equal?(x=50, y=w57) -> (x = y?=w52:bool)
          n19 = xnode "Read/Write Control"("FPGA VI Reference In"=w59, "error in"=w50) -> ("FPGA VI Reference Out"=w55:refnum<k20>, "error out"=w54:errorcluster, "Init Done"=w51)
          n20 = Or(x=w51, y=w52) -> (x .or. y?=w53:bool)
          n21 = Wait Until Next ms Multiple(millisecond multiple=u32 100) -> ()  [unwired: 1 out]
        }
        n22 = case shown="False" w29 {
          tunnel: [w45 w49] -> w24
          tunnel: w28 -> [w45 w49]
          tunnel: w27 -> [w44 w47]
          tunnel: [w44 w48] -> w23
          frame False {
          }
          frame True {
            # "InitDone timeout"
            n23 = Merge Errors(w47, errorcluster {"status"=TRUE, "code"=-1, "source"="The IO Module CLIP was not ready. If you are using any external clocks, make sure they are connected and within the supported specifications."} ("error in")) -> (w48:errorcluster)
          }
        }
        n24 = while {
          tunnel: [w81] -> w43
          tunnel: "Num Samples" -> [w72]
          tunnel: w24 -> [w79]
          shift-right: [w75] -> _
          shift-left: u32 0 ("Timeout (ms)") -> [w74]
          tunnel: "Num Records" -> [w73]
          shift-right: [w69] -> w31
          shift-left: T3 [] -> [w70]
          shift-right: [w80] -> w42
          shift-left: w23 -> [w68]
          shift-right: [w60] -> _
          shift-left: u32 0 ("Timeout (ms)") -> [w61]
          stop <- w65 stop-if-true
          n25 = Decrement(x=w73) -> (x-1=w71:u32)
          n26 = xnode "Read/Write Control"("FPGA VI Reference In"=w79, "error in"=w68) -> ("FPGA VI Reference Out"=w76:refnum<k20>, "error out"=w63:errorcluster, "Records Available"=w78, "FIFO Overflow"=w64)
          n27 = Unbundle By Name(w68) -> ("status"=w67:bool)
          n28 = Equal?(x=w74, y=w71) -> (x = y?=w66:bool)
          n29 = Or(x=w66, y=w67) -> (x .or. y?=w65:bool)
          n30 = Greater Than 0?(x=w78) -> (x > 0?=w77:bool)
          n31 = case shown="False" w64 {
            tunnel: w63 -> [w82 w84]
            tunnel: [w82 w83] -> w62
            frame False {
            }
            frame True {
              n32 = Merge Errors(w84, errorcluster {"status"=TRUE, "code"=-1, "source"="The DMA FIFO has overflown.  Try reducing number of records and record size."} ("error in")) -> (w83:errorcluster)
            }
          }
          n33 = case shown="True" w77 {
            tunnel: [w95 w114] -> w81
            tunnel: [w87 w113] -> w80
            tunnel: w72 -> [_ w112]
            tunnel: w76 -> [w95 w110]
            tunnel: w62 -> [w88 w109]
            tunnel: [w94 w107] -> w75
            tunnel: w74 -> [w94 w108]
            tunnel: w70 -> [w93 w104]
            tunnel: [w93 w103] -> w69
            tunnel: w61 -> [w92 _]
            tunnel: [w86 u32 0 ("Timeout (ms)")] -> w60
            frame False {
              n34 = Increment(x=w92) -> (x+1=w86:u32)
              n35 = Equal?(x=w86, y="Timeout (sec)") -> (x = y?=w90:bool)
              n36 = case shown="True" w90 {
                tunnel: w88 -> [w96 w98]
                tunnel: [w96 w99] -> w87
                frame False {
                }
                frame True {
                  n37 = Merge Errors(w98, errorcluster {"status"=TRUE, "code"=-1, "source"="Maximum time exceeded before the acquisition completed.  If using a digital trigger, check that it is properly supplied."} ("error in")) -> (w99:errorcluster)
                }
              }
              n38 = Wait (ms)(milliseconds to wait=u32 1000) -> ()  [unwired: 1 out]
            }
            frame True {
              # "7."
              n39 = xnode "Invoke Method"("FPGA VI Reference In"=w110, "error in"=w109, "Number of Elements"=w112, "Timeout (ms)"=5000) -> ("FPGA VI Reference Out"=w114:refnum<k20>, "error out"=w113:errorcluster, "Data"=w105:void[])  [unwired: 1 out]
              n40 = Increment(x=w108) -> (x+1=w107:u32)
              n41 = Bundle("absoluteInitialX"=0.0, "xIncrement"=1.0, "Data"=w105) -> (w102:T4)  [unwired: 1 out]
              n42 = Build Array (concatenate)(w104, w102) -> (w103:T3)
            }
          }
        }
      }
      frame True {
        # "The IO Module was not present, powered, or the IO were not enabled.\nVerify the NI 5751 is securly connected and try again."
        n43 = Merge Errors(w118, errorcluster {"status"=TRUE, "code"=-1, "source"="The IO Module was not present, powered, or the IO were not enabled.  Verify the NI 5751 is securly connected and try again."} ("error in")) -> (w117:errorcluster)
      }
    }
    "Wfm Graph" <- w14
    n44 = xnode "Close FPGA VI Reference"("FPGA VI Reference In"=w15, "error in"=w17) -> ("error out"=w18:errorcluster)
    n45 = Array Size(array=w14) -> (size(s)=→"Records Displayed":i32)
    n46 = call <vilib>:"Simple Error Handler.vi"("error in (no error)"=w18) -> ("error out"=w6:errorcluster)  [unwired: 1 in, 7 out]
    "error out" <- w6
    n47 = Unbundle By Name(w6) -> ("status"=w3:bool)
    n48 = Or(x=w3, y="stop") -> (x .or. y?=w5:bool)
  }
